vi "set_min_max.vi"(9 "max_value":dbl, 10 "min_value":dbl, 11 "array_in":dbl[][](array[numeric])) -> (3 "array_out":u16[][](array[numeric]))   [LabVIEW 2019]
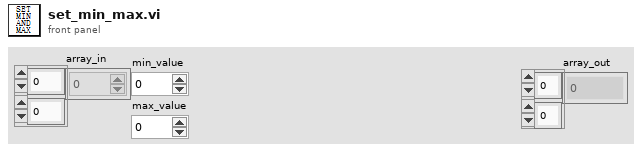
[diagram p1: front panel]
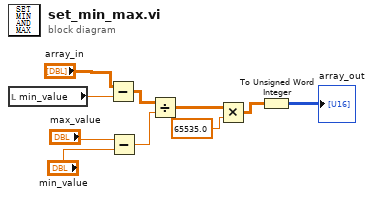
[diagram p0: block diagram]
diagram:
  n1 = local read "min_value"() -> (w9:dbl)
  n2 = Subtract(x="array_in", y=w9) -> (x-y=w7:dbl[][])
  n3 = Subtract(x="max_value", y="min_value") -> (x-y=w4:dbl)
  n4 = Divide(x=w7, y=w4) -> (x/y=w3:dbl[][])
  n5 = Multiply(x=w3, y=65535.0) -> (x*y=w1:dbl[][])
  n6 = To Unsigned Word Integer(number=w1) -> (unsigned 16bit integer=→"array_out":u16[][])
